vi "TektronixDPO4000OscilloScope.vi"() -> ()   [LabVIEW 2021]
uses:
  lib/Hardware/TextControlledInstrum/IOQueuePacket.ctl
  lib/Hardware/TextControlledInstrum/ControlToCommandMulti.vi
  lib/Hardware/TextControlledInstrum/TextControlledInstrum.lvlib
panel:
  in  "Pause":bool
  in  "Clear":bool
  in  "Enable":bool
  in  "Log":string
  in  "Force":bool
  out "Updating":bool
  in  "Single":bool
  in  "Start/Stop":bool
  in  "Clear Menu":bool
  in  "Acquire":T1 {"Num Average" items=["2"=2, "4"=4, "8"=8, "16"=16, "32"=32, "64"=64, "128"=128, "256"=256, "512"=512]}
  in  "Trigger":T2 {"Holdoff" format="%#_6p"; "Level (V)" format="%#_6p"}
  in  "Horizontal":T3={"Scale / Div"=1e-09, "Mode"=enum."Position", "Delay"=0.0, "Position"=0.0, "Position Zero"=FALSE, "Sampling Rate (Hz)"=0.0, "Record Length"=0} {"Delay" format="%#_6p"; "Position" format="%#_6p"; "Scale / Div" items=["1n", "2n", "4n", "10n", "20n", "40n", "100n", "200n", "400n", "1u", "2u", "4u", "10u", "20u", "40u", "100u", "200u", "400u", "1m", "2m", "4m", "10m", "20m", "40m", "100m", "200m", "400m", "1", "2", "4", "10", "20", "40", "100", "200", "400", "1k"]; "Sampling Rate (Hz)" format="%#_6p"; "Record Length" items=["1k"=1000, "10k"=10000, "100k"=100000, "1M"=1000000, "5M"=5000000, "10M"=10000000]}
  in  "CH4 Enabled":bool
  in  "CH3 Enabled":bool
  in  "CH2 Enabled":bool
  in  "CH1 Enabled":bool
  in  "CH4":T4 {"Deskew" format="%#_6p"; "Termination" items=["50 Ohm"=50.0, "1 MOhm"=1000000.0]; "Offset" format="%#_6p"; "Position / Div" min=-5.0 max=5.0 step=0.1; "Scale / Div" items=["0.1 mV"=0.0001, "0.2 mV"=0.0002, "0.5 mV"=0.0005, "1 mV"=0.001, "2 mV"=0.002, "5 mV"=0.005, "10 mV"=0.01, "20 mV"=0.02, "50 mV"=0.05, "0.1 V"=0.1, "0.2 V"=0.2, "0.5 V"=0.5, "1 V"=1.0, "2 V"=2.0, "5 V"=5.0, "10 V"=10.0]; "Bandwidth" items=["20 MHz"=20000000.0, "250 MHz"=250000000.0, "Full"=500000000.0]}
  in  "CH3":T4 {"Deskew" format="%#_6p"; "Termination" items=["50 Ohm"=50.0, "1 MOhm"=1000000.0]; "Offset" format="%#_6p"; "Position / Div" min=-5.0 max=5.0 step=0.1; "Scale / Div" items=["0.1 mV"=0.0001, "0.2 mV"=0.0002, "0.5 mV"=0.0005, "1 mV"=0.001, "2 mV"=0.002, "5 mV"=0.005, "10 mV"=0.01, "20 mV"=0.02, "50 mV"=0.05, "0.1 V"=0.1, "0.2 V"=0.2, "0.5 V"=0.5, "1 V"=1.0, "2 V"=2.0, "5 V"=5.0, "10 V"=10.0]; "Bandwidth" items=["20 MHz"=20000000.0, "250 MHz"=250000000.0, "Full"=500000000.0]}
  in  "CH2":T4 {"Deskew" format="%#_6p"; "Termination" items=["50 Ohm"=50.0, "1 MOhm"=1000000.0]; "Offset" format="%#_6p"; "Position / Div" min=-5.0 max=5.0 step=0.1; "Scale / Div" items=["0.1 mV"=0.0001, "0.2 mV"=0.0002, "0.5 mV"=0.0005, "1 mV"=0.001, "2 mV"=0.002, "5 mV"=0.005, "10 mV"=0.01, "20 mV"=0.02, "50 mV"=0.05, "0.1 V"=0.1, "0.2 V"=0.2, "0.5 V"=0.5, "1 V"=1.0, "2 V"=2.0, "5 V"=5.0, "10 V"=10.0]; "Bandwidth" items=["20 MHz"=20000000.0, "250 MHz"=250000000.0, "Full"=500000000.0]}
  in  "CH1":T4 {"Deskew" format="%#_6p"; "Termination" items=["50 Ohm"=50.0, "1 MOhm"=1000000.0]; "Offset" format="%#_6p"; "Position / Div" min=-5.0 max=5.0 step=0.1; "Scale / Div" items=["0.1 mV"=0.0001, "0.2 mV"=0.0002, "0.5 mV"=0.0005, "1 mV"=0.001, "2 mV"=0.002, "5 mV"=0.005, "10 mV"=0.01, "20 mV"=0.02, "50 mV"=0.05, "0.1 V"=0.1, "0.2 V"=0.2, "0.5 V"=0.5, "1 V"=1.0, "2 V"=2.0, "5 V"=5.0, "10 V"=10.0]; "Bandwidth" items=["20 MHz"=20000000.0, "250 MHz"=250000000.0, "Full"=500000000.0]}
  in  "VISA resource name":refnum<visa-resource-name>
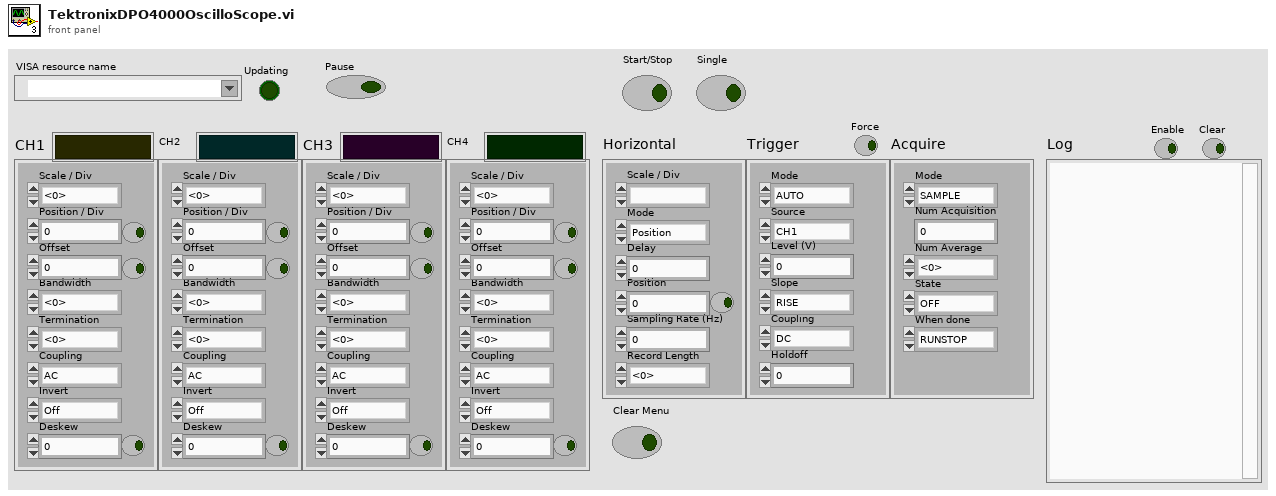
[diagram p1: front panel]
types:
  T1 = cluster{"Mode":enum16{"SAMPLE", "PEAKDETECT", "HIRES", "AVERAGE", "ENVELOPE"}, "Num Acquisition":u32, "Num Average":u16, "State":enum16{"OFF", "ON", "RUN", "STOP"}, "When done":enum16{"RUNSTOP", "SEQUENCE"}}
  T2 = cluster{"Mode":enum16{"AUTO", "NORMAL"}, "Source":enum16{"CH1", "CH2", "CH3", "CH4", "EXT", "LINE", "AUX"}, "Level (V)":dbl, "Slope":enum16{"RISE", "FALL"}, "Coupling":enum16{"DC", "HFREJ", "LFREJ", "NOISEREJ"}, "Holdoff":dbl}
  T3 = cluster{"Scale / Div":ext, "Mode":enum16{"Position", "Delay"}, "Delay":dbl, "Position":dbl, "Position Zero":bool, "Sampling Rate (Hz)":dbl, "Record Length":u32}
  T4 = cluster{"Query Only":string, "Scale / Div":dbl, "Position / Div":dbl, "Position Zero":bool, "Offset":dbl, "Offset Zero":bool, "Bandwidth":dbl, "Termination":dbl, "Coupling":enum16{"AC", "DC", "GND"}, "Invert":enum16{"Off", "On"}, "Deskew":dbl, "Deskew Zero 2":bool}
  T5 = typedef "TextControlledInstrum.lvlib/IOQueuePacket.ctl" = cluster{"Operation":enum16{"read", "write", "reserved2", "reserved3", "reserved4", "reserved5", "reserved6", "reserved7"}, "Data":string, "Queue":refnum<queue>}
  T6 = enum16{"read", "write", "reserved2", "reserved3", "reserved4", "reserved5", "reserved6", "reserved7"}
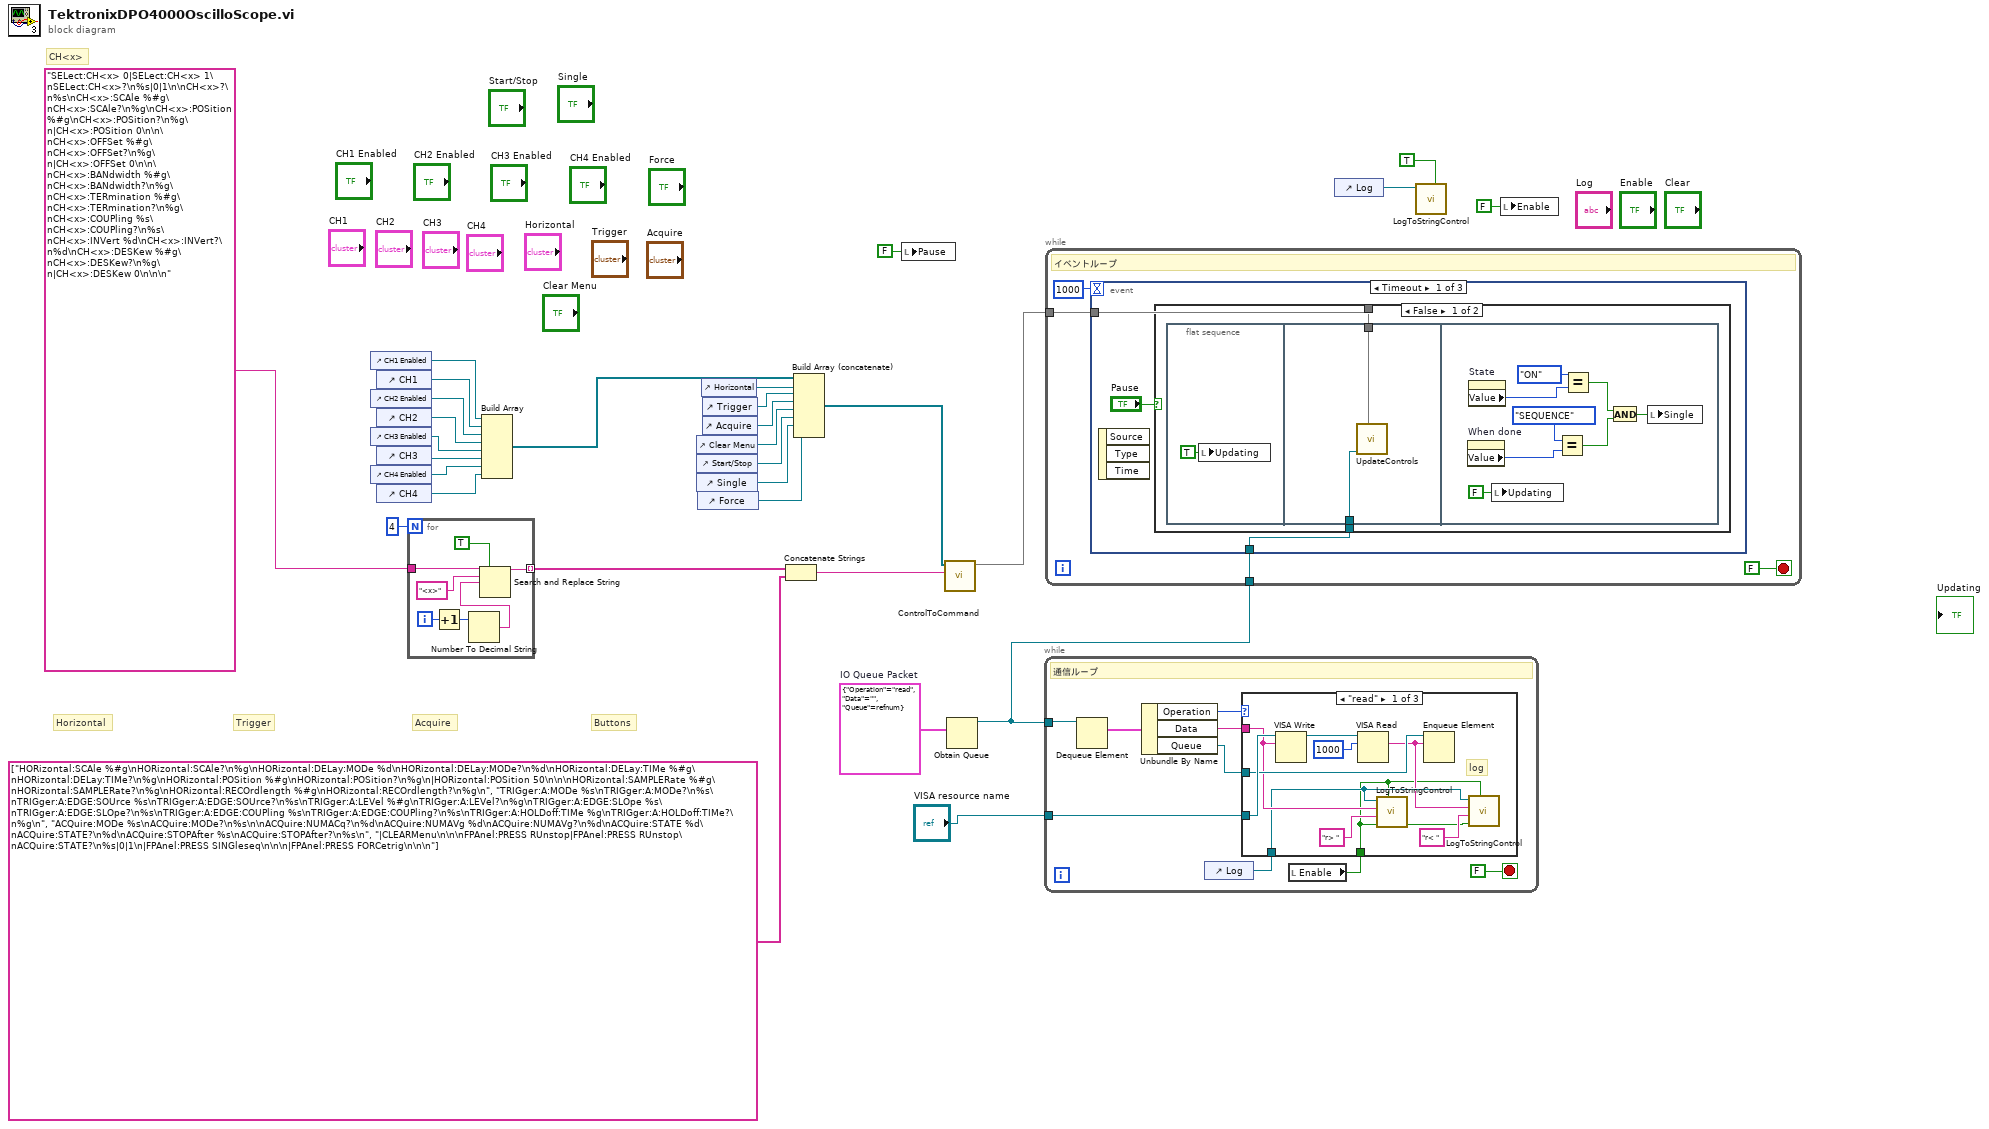
[diagram p0: block diagram]
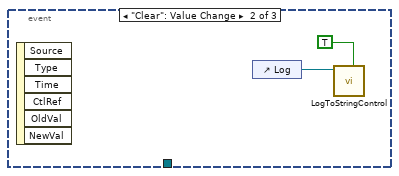
[diagram p3: hidden frame]
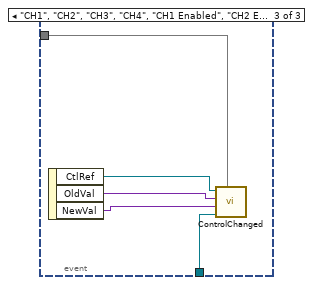
[diagram p4: hidden frame]
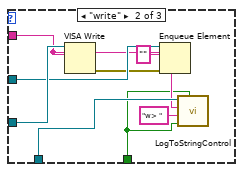
[diagram p5: hidden frame]
diagram:
  w28 = T5 {"Operation"=enum."read", "Data"="", "Queue"=refnum}  # IO Queue Packet
  # "Buttons"
  # "Acquire"
  # "Trigger"
  # "Horizontal"
  # "CH<x>"
  n1 = control-ref of="CH1 Enabled"() -> (w25:refnum<vi>)
  n2 = control-ref of="CH2 Enabled"() -> (w23:refnum<vi>)
  n3 = control-ref of="CH3 Enabled"() -> (w21:refnum<vi>)
  n4 = control-ref of="CH4 Enabled"() -> (w19:refnum<vi>)
  n5 = control-ref of="CH1"() -> (w24:refnum<vi>)
  n6 = control-ref of="CH2"() -> (w22:refnum<vi>)
  n7 = control-ref of="CH3"() -> (w20:refnum<vi>)
  n8 = control-ref of="CH4"() -> (w18:refnum<vi>)
  n9 = for {
    N: 4 -> [_]
    tunnel: "SELect:CH<x> 0|SELect:CH<x> 1\nSELect:CH<x>?\n%s|0|1\n\nCH<x>?\n%s\nCH<x>:SCAle %#g\nCH<x>:SCAle?\n%g\nCH<x>:POSition %#g\nCH<x>:POSition?\n%g\n|CH<x>:POSition 0\n\n\nCH<x>:OFFSet %#g\nCH<x>:OFFSet?\n%g\n|CH<x>:OFFSet 0\n\n\nCH<x>:BANdwidth %#g\nCH<x>:BANdwidth?\n%g\nCH<x>:TERmination %#g\nCH<x>:TERmination?\n%g\nCH<x>:COUPling %s\nCH<x>:COUPling?\n%s\nCH<x>:INVert %d\nCH<x>:INVert?\n%d\nCH<x>:DESKew %#g\nCH<x>:DESKew?\n%g\n|CH<x>:DESKew 0\n\n\n" -> [w37]
    tunnel: [w34] -> w29 mode=indexing
    i -> [w33]
    n10 = Increment(x=w33) -> (x+1=w32:i32)
    n11 = Number To Decimal String(number=w32) -> (decimal integer string=w31:string)  [unwired: 1 in]
    n12 = Search and Replace String(replace all?=TRUE ("replace all? (F)"), input string=w37, search string="<x>", replace string=w31) -> (result string=w34:string)  [unwired: 4 in, 3 out]
  }
  n13 = Build Array(w25, w24, w23, w22, w21, w20, w19, w18) -> (w27:refnum<vi>[])
  n14 = control-ref of="Clear Menu"() -> (w12:refnum<vi>)
  n15 = control-ref of="Start/Stop"() -> (w10:refnum<vi>)
  n16 = control-ref of="Single"() -> (w9:refnum<vi>)
  n17 = control-ref of="Force"() -> (w6:refnum<vi>)
  n18 = control-ref of="Horizontal"() -> (w16:refnum<vi>)
  n19 = control-ref of="Trigger"() -> (w14:refnum<vi>)
  n20 = control-ref of="Acquire"() -> (w13:refnum<vi>)
  n21 = Concatenate Strings(w29, string[] ["HORizontal:SCAle %#g\nHORizontal:SCAle?\n%g\nHORizontal:DELay:MODe %d\nHORizontal:DELay:MODe?\n%d\nHORizontal:DELay:TIMe %#g\nHORizontal:DELay:TIMe?\n%g\nHORizontal:POSition %#g\nHORizontal:POSition?\n%g\n|HORizontal:POSition 50\n\n\nHORizontal:SAMPLERate %#g\nHORizontal:SAMPLERate?\n%g\nHORizontal:RECOrdlength %#g\nHORizontal:RECOrdlength?\n%g\n", "TRIGger:A:MODe %s\nTRIGger:A:MODe?\n%s\nTRIGger:A:EDGE:SOUrce %s\nTRIGger:A:EDGE:SOUrce?\n%s\nTRIGger:A:LEVel %#g\nTRIGger:A:LEVel?\n%g\nTRIGger:A:EDGE:SLOpe %s\nTRIGger:A:EDGE:SLOpe?\n%s\nTRIGger:A:EDGE:COUPling %s\nTRIGger:A:EDGE:COUPling?\n%s\nTRIGger:A:HOLDoff:TIMe %g\nTRIGger:A:HOLDoff:TIMe?\n%g\n", "ACQuire:MODe %s\nACQuire:MODe?\n%s\n\nACQuire:NUMACq?\n%d\nACQuire:NUMAVg %d\nACQuire:NUMAVg?\n%d\nACQuire:STATE %d\nACQuire:STATE?\n%d\nACQuire:STOPAfter %s\nACQuire:STOPAfter?\n%s\n", "|CLEARMenu\n\n\nFPAnel:PRESS RUnstop|FPAnel:PRESS RUnstop\nACQuire:STATE?\n%s|0|1\n|FPAnel:PRESS SINGleseq\n\n\n|FPAnel:PRESS FORCetrig\n\n\n"]) -> (w15:string)
  n22 = Build Array (concatenate)(w27, w16, w14, w13, w12, w10, w9, w6) -> (w17:refnum<vi>[])
  n23 = local write "Pause"(FALSE ("Pause")) -> ()
  n24 = call-poly "ControlToCommand.vi"("SetGetCommands"=w15, "Control Array"=w17) -> ("ControlToCommand"=w8:map{refnum<vi>, string[]})  [unwired: 9 in]
  n25 = Obtain Queue(element data type=w28) -> (queue out=w7:refnum<queue>)  [unwired: 4 in, 2 out]
  n26 = while {
    tunnel: w7 -> [w46]
    tunnel: "VISA resource name" -> [w38]
    stop <- FALSE stop-if-true
    # "通信ループ"
    n27 = Dequeue Element(queue=w46) -> (element=w45:T5)  [unwired: 2 in, 3 out]
    n28 = Unbundle By Name(w45) -> ("Operation"=w44:T6, "Data"=w43:string, "Queue"=w42:refnum<queue>)
    n29 = control-ref of="Log"() -> (w40:refnum<vi>)
    n30 = local read "Enable"() -> (w39:bool)
    n31 = case shown="\"read\"" w44 {
      tunnel: w43 -> [w52 w58 _]
      tunnel: w38 -> [w54 w64 _]
      tunnel: w42 -> [w53 w63 _]
      tunnel: w40 -> [w49 w59 _]
      tunnel: w39 -> [w47 w57 _]
      frame "read" {
        # "log"
        n32 = VISA Write(VISA resource name=w54, write buffer=w52) -> (VISA resource name out=w56:refnum<visa-resource-name>)  [unwired: 1 in, 2 out]
        n33 = VISA Read(VISA resource name=w56, byte count=u32 1000) -> (read buffer=w48:string)  [unwired: 1 in, 3 out]
        n34 = call "LogToStringControl.vi"("Enable"=w47, "Time Stamp (T/F or Format)"=w47, "Prefix (\"\")"="r> " ("Prefix (\"\")"), "Log Text (\"\")"=w52, "String Ref"=w49) -> ()  [unwired: 6 in, 1 out]
        n35 = Enqueue Element(queue=w53, element=w48) -> ()  [unwired: 2 in, 3 out]
        n36 = call "LogToStringControl.vi"("Enable"=w47, "Time Stamp (T/F or Format)"=w47, "Prefix (\"\")"="r< " ("Prefix (\"\")"), "Log Text (\"\")"=w48, "String Ref"=w49) -> ()  [unwired: 6 in, 1 out]
      }
      frame "write" {
        n37 = VISA Write(VISA resource name=w64, write buffer=w58) -> (error out=w61:errorcluster)  [unwired: 1 in, 2 out]
        n38 = Enqueue Element(queue=w63, element="", error in (no error)=w61) -> ()  [unwired: 1 in, 3 out]
        n39 = call "LogToStringControl.vi"("Enable"=w57, "Time Stamp (T/F or Format)"=w57, "Prefix (\"\")"="w> " ("Prefix (\"\")"), "Log Text (\"\")"=w58, "String Ref"=w59) -> ()  [unwired: 6 in, 1 out]
      }
      frame Default {
      }
    }
  }
  n40 = while {
    tunnel: w8 -> [w67]
    tunnel: w7 -> [w66]
    stop <- FALSE stop-if-true
    # "イベントループ"
    n41 = event shown="[0] Timeout" {
      selector: _ -> [_ _ _]
      dyn-events: _ -> [_ _ _]
      timeout: 1000 -> [_ _ _]
      tunnel: w67 -> [w71 _ w87]
      tunnel: w66 -> [w70 _ w91]
      event Timeout {
        n42 = event-data() -> ()  [unwired: 1 in, 3 out]
        n43 = case shown="False" "Pause" {
          tunnel: w71 -> [w73 _]
          tunnel: w70 -> [w72 _]
          frame False {
            n44 = flat-sequence {
              tunnel: w73 -> [w76]
              tunnel: w72 -> [w75]
              frame #0 {
                n45 = local write "Updating"(TRUE ("Updating")) -> ()
              }
              frame #1 {
                n46 = call "UpdateControls.vi"("ControlToCommand"=w76, "IO Queue"=w75) -> ()  [unwired: 9 in, 1 out]
              }
              frame #2 {
                n47 = property on="When done" class="Enum (strict)"() -> ("Value"=w80:enum16{"RUNSTOP", "SEQUENCE"})  [unwired: 2 in, 2 out]
                n48 = property on="State" class="Enum (strict)"() -> ("Value"=w82:enum16{"OFF", "ON", "RUN", "STOP"})  [unwired: 2 in, 2 out]
                n49 = local write "Updating"(FALSE ("Updating")) -> ()
                n50 = Equal?(x=enum16{"RUNSTOP", "SEQUENCE"}."SEQUENCE" ("Value"), y=w80) -> (x = y?=w78:bool)
                n51 = Equal?(x=enum16{"OFF", "ON", "RUN", "STOP"}."ON" ("Value"), y=w82) -> (x = y?=w79:bool)
                n52 = And(x=w79, y=w78) -> (x .and. y?=w77:bool)
                n53 = local write "Single"(w77) -> ()
              }
            }
          }
          frame True {
          }
        }
      }
      event "Clear": Value Change {
        n54 = event-data() -> ()  [unwired: 1 in, 6 out]
        n55 = control-ref of="Log"() -> (w86:refnum<vi>)
        n56 = call "LogToStringControl.vi"("Clear"=TRUE, "String Ref"=w86) -> ()  [unwired: 9 in, 1 out]
      }
      event "CH1", "CH2", "CH3", "CH4", "CH1 Enabled", "CH2 Enabled", "CH3 Enabled", "CH4 Enabled", "Horizontal", "Trigger", "Acquire", "Clear Menu", "Start/Stop", "Single", "Force": Value Change {
        n57 = event-data() -> ("CtlRef"=w88:refnum<vi>, "OldVal"=w89:variant, "NewVal"=w90:variant)  [unwired: 1 in]
        n58 = call "ControlChanged.vi"("ControlToCommand"=w87, "IO Queue"=w91, "NewVal"=w90, "OldVal"=w89, "CtlRef"=w88) -> ()  [unwired: 6 in, 1 out]
      }
    }
  }
  n59 = control-ref of="Log"() -> (w3:refnum<vi>)
  n60 = call "LogToStringControl.vi"("Clear"=TRUE, "String Ref"=w3) -> ()  [unwired: 9 in, 1 out]
  n61 = local write "Enable"(FALSE ("Enable")) -> ()
